vi "fix_relativepath.vi"(10 "relative_path":string) -> (2 "fixed_relative_path":string)   [LabVIEW 2013]
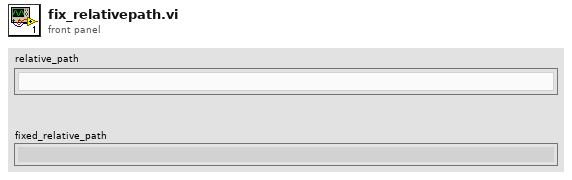
[diagram p1: front panel]
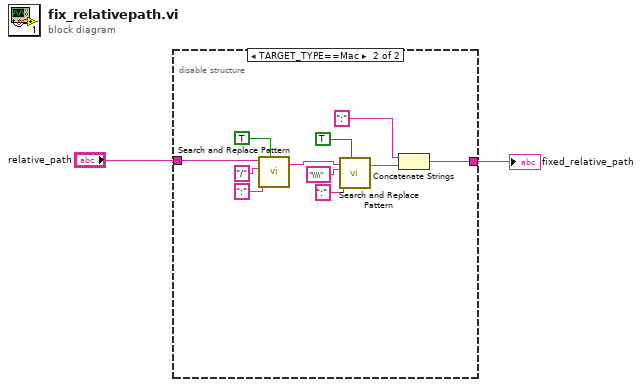
[diagram p0: block diagram]
diagram:
  n1 = disable-structure shown="TARGET_TYPE==Mac" {
    disable-tunnel: "relative_path" -> [w3 w11]
    disable-tunnel: [w3 w9] -> w1
    frame condition #0 {
    }
    frame condition #1 (active) {
      n2 = call <vilib>:"Search and Replace Pattern.vi"("string"=w11, "regular expression (\"\")"="/" ("regular expression (\"\")"), "replace string (\"\")"=":" ("replace string (\"\")"), "replace all? (F)"=TRUE) -> ("result string"=w5:string)  [unwired: 1 in, 1 out]
      n3 = call <vilib>:"Search and Replace Pattern.vi"("string"=w5, "regular expression (\"\")"="\\\\" ("regular expression (\"\")"), "replace string (\"\")"=":" ("replace string (\"\")"), "replace all? (F)"=TRUE) -> ("result string"=w4:string)  [unwired: 1 in, 1 out]
      n4 = Concatenate Strings(":" ("replace string (\"\")"), w4) -> (w9:string)
    }
  }
  "fixed_relative_path" <- w1
